vi "MoveOneStep.vi"(8 "error in (no error)":errorcluster, 11 "Snake in":refnum<class "Snake.lvclass">) -> (0 "error out":errorcluster, 3 "Snake out":refnum<class "Snake.lvclass">)   [LabVIEW 2018, in "Snake.lvclass"]
uses:
  Snake.lvclass
  Snake.lvclass/Snake.ctl
  BodyCell/SnakeBodyCell.lvclass
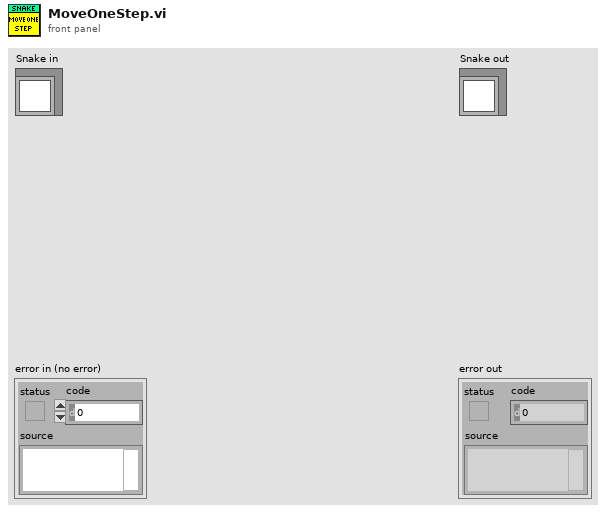
[diagram p1: front panel]
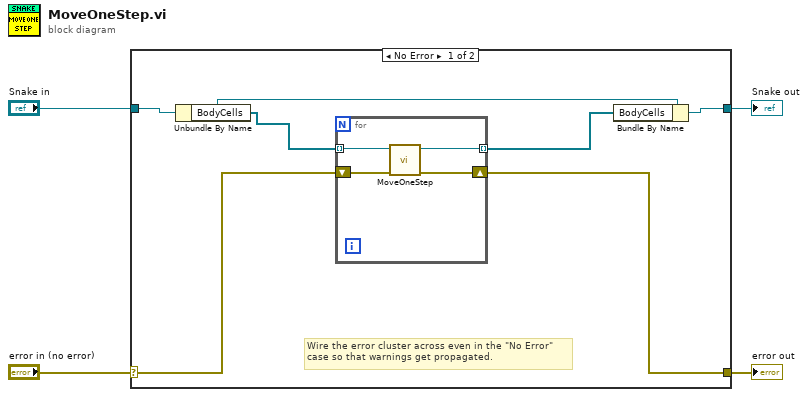
[diagram p0: block diagram]
diagram:
  n1 = case shown="No Error" "error in (no error)" {
    selector: "error in (no error)" -> [w6 w16]
    tunnel: [w5 w16] -> w3
    tunnel: [w9 w15] -> w1
    tunnel: "Snake in" -> [w10 w15]
    frame No Error {
      # "Wire the error cluster across even in the \"No Error\"\ncase so that warnings get propagated."
      n2 = Unbundle By Name(w10) -> ("BodyCells"=w8:refnum<class "SnakeBodyCell.lvclass">[])
      n3 = for {
        tunnel: w8 -> [w14] mode=indexing
        tunnel: [w13] -> w7 mode=indexing
        shift-right: [w11] -> w5
        shift-left: w6 -> [w12]
        n4 = call "MoveOneStep.vi"("error in (no error)"=w12, "SnakeBodyUnit in"=w14) -> ("error out"=w11:errorcluster, "SnakeBodyUnit out"=w13:refnum<class "SnakeBodyCell.lvclass">)  [unwired: 8 in]
      }
      n5 = Bundle By Name(cluster=w10, "BodyCells"=w7) -> (w9:refnum<class "Snake.lvclass">)
    }
    frame Error {
    }
  }
  "error out" <- w3
  "Snake out" <- w1
